vi "Generate Get Connections Error Message.vi"(8 "error in":errorcluster, 9 "instrument type id":string, 10 "site":i32, 11 "pin or relay names":string) -> (0 "error out":errorcluster, 3 "error string":string)   [LabVIEW 2020, in "MeasurementLink Session Management.lvlib" / "Session Reservation.lvclass"]
uses:
  Session Reservation.lvclass
  Session Reservation.lvclass/Session Reservation.ctl
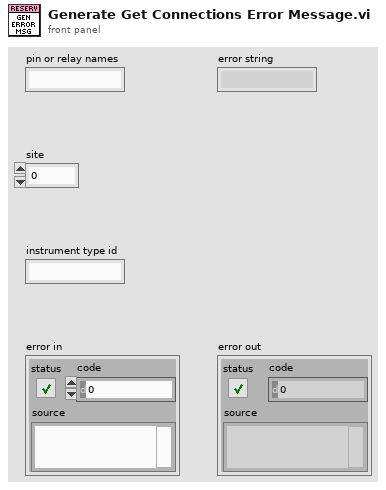
[diagram p1: front panel]
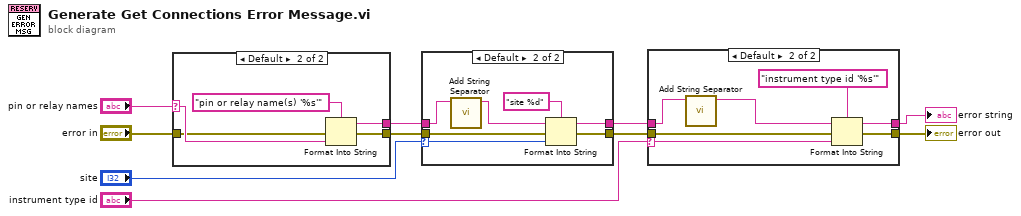
[diagram p0: block diagram]
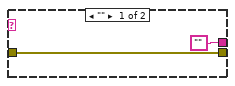
[diagram p2: hidden frame]
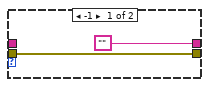
[diagram p4: hidden frame]
diagram:
  n1 = case shown="Default" "pin or relay names" {
    selector: "pin or relay names" -> [_ w15]
    tunnel: ["" w17] -> w7
    tunnel: "error in" -> [w11 w14]
    tunnel: [w11 w13] -> w8
    frame "" {
    }
    frame Default {
      n2 = Format Into String(format string="pin or relay name(s) '%s'", error in=w14, w15) -> (resulting string=w17:string, error out=w13:errorcluster)  [unwired: 1 in]
    }
  }
  n3 = case shown="Default" "site" {
    selector: "site" -> [_ w24]
    tunnel: ["" w26] -> w4
    tunnel: w8 -> [w18 w23]
    tunnel: [w18 w22] -> w1
    tunnel: w7 -> [_ w21]
    frame -1 {
    }
    frame Default {
      n4 = call "Add String Separator.vi"("string in"=w21) -> ("string out"=w20:string)  [unwired: 10 in]
      n5 = Format Into String(format string="site %d", initial string=w20, error in=w23, w24) -> (resulting string=w26:string, error out=w22:errorcluster)
    }
  }
  n6 = case shown="Default" "instrument type id" {
    selector: "instrument type id" -> [_ w31]
    tunnel: [w27 w35] -> w10
    tunnel: w1 -> [w28 w33]
    tunnel: [w28 w32] -> w3
    tunnel: w4 -> [w27 w29]
    frame "" {
    }
    frame Default {
      n7 = call "Add String Separator.vi"("string in"=w29) -> ("string out"=w30:string)  [unwired: 10 in]
      n8 = Format Into String(format string="instrument type id '%s'", initial string=w30, error in=w33, w31) -> (resulting string=w35:string, error out=w32:errorcluster)
    }
  }
  "error string" <- w10
  "error out" <- w3
